vi "UT_Main.vi"(8 "error in":errorcluster, 10 "Report Path":path, 11 "Interactive":bool) -> (0 "error out":errorcluster)   [LabVIEW 2017]
doc: "Main VI for all unit tests. All unit test VIs are hierachically called from this VI."
uses:
  <vilib>/addons/_JKI Toolkits/Caraya/classes/Test Suite/Test Suite.lvclass
  UT_LogRecord/UT_LogRecord.lvlib
  UT_Helper/UT_Helper.lvlib
  UT_Handler/UT_UserEventHandler/UT_UserEventHandler.lvlib
  UT_Formatter/UT_Formatter.lvlib
  UT_Formatter/UT_JSONLFormatter/UT_JSONLFormatter.lvlib
  UT_Handler/UT_FileHandler/UT_FileHandler.lvlib
  <vilib>/addons/_JKI Toolkits/Caraya/classes/Test Suite/Define Test Suite (SimpleText Report).vi
  UT_Formatter/UT_LokiJsonFormatter/UT_LokiJsonFormatter.lvlib
  UT_Handler/UT_LokiHandler/UT_LokiHandler.lvlib
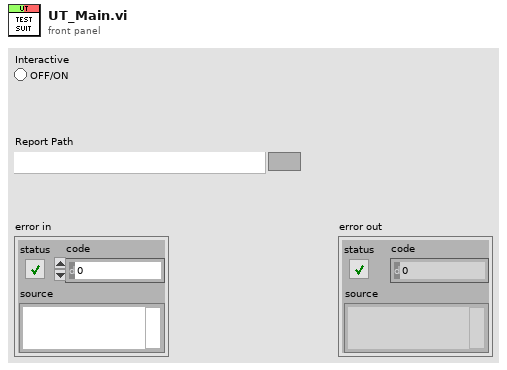
[diagram p1: front panel]
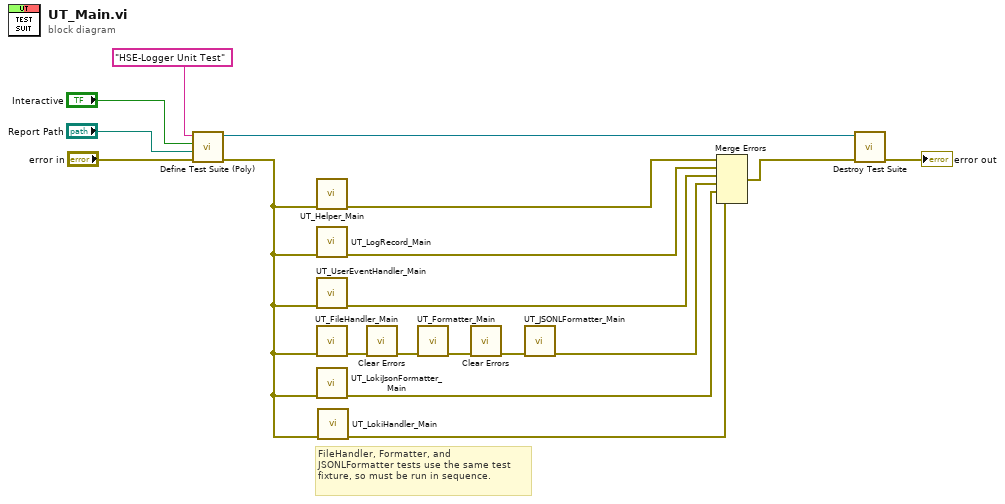
[diagram p0: block diagram]
diagram:
  # "FileHandler, Formatter, and JSONLFormatter tests use the same test fixture, so must be run in sequence."
  n1 = call-poly <vilib>:"Define Test Suite (Poly).vi"("error in (no error)"="error in", "Report Path"="Report Path", "Interactive"="Interactive", "Label (VI Title)"="HSE-Logger Unit Test") -> ("error out"=w3:errorcluster, "Test Suite"=w5:refnum<class "Test Suite.lvclass">)  [unwired: 5 in, 1 out]
  n2 = call "UT_Helper_Main.vi"("error in"=w3) -> ("error out"=w13:errorcluster)  [unwired: 10 in]
  n3 = call "UT_LogRecord_Main.vi"("error in"=w3) -> ("error out"=w14:errorcluster)  [unwired: 10 in]
  n4 = call "UT_UserEventHandler_Main.vi"("error in (no error)"=w3) -> ("error out"=w15:errorcluster)  [unwired: 10 in]
  n5 = call "UT_FileHandler_Main.vi"("error in"=w3) -> ("error out"=w12:errorcluster)  [unwired: 10 in]
  n6 = call "UT_LokiJsonFormatter_Main.vi"("error in"=w3) -> ("error out"=w2:errorcluster)  [unwired: 10 in]
  n7 = call "UT_LokiHandler_Main.vi"("error in (no error)"=w3) -> ("error out"=w1:errorcluster)  [unwired: 10 in]
  n8 = call <vilib>:"Clear Errors.vi"("error in (no error)"=w12) -> ("error out"=w9:errorcluster)  [unwired: 5 in, 1 out]
  n9 = call "UT_Formatter_Main.vi"("error in"=w9) -> ("error out"=w11:errorcluster)  [unwired: 10 in]
  n10 = call <vilib>:"Clear Errors.vi"("error in (no error)"=w11) -> ("error out"=w8:errorcluster)  [unwired: 5 in, 1 out]
  n11 = call "UT_JSONLFormatter_Main.vi"("error in"=w8) -> ("error out"=w10:errorcluster)  [unwired: 10 in]
  n12 = Merge Errors(w13, w14, w15, w10, w2, w1) -> (w16:errorcluster)
  n13 = call-dynamic "Destroy Test Suite.vi"("error in (no error)"=w16, "Test Suite in"=w5) -> ("error out"=→"error out":errorcluster)  [unwired: 8 in, 1 out]
